vi "Calculate Mean Free Path.vi"(8 "error in (no error)":errorcluster, 11 "Gas Properties in":refnum<class "Gas Properties.lvclass">) -> (0 "error out":errorcluster, 2 "l (mm)":dbl, 3 "Gas Properties out":refnum<class "Gas Properties.lvclass">)   [LabVIEW 2015, in "Gas Properties.lvclass"]
uses:
  Gas Properties.lvclass
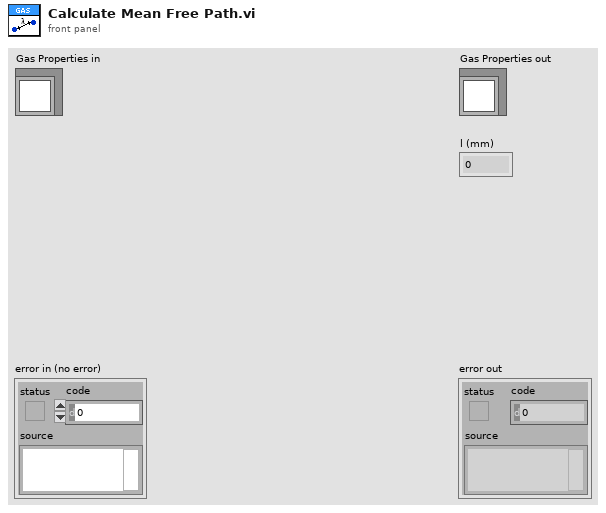
[diagram p1: front panel]
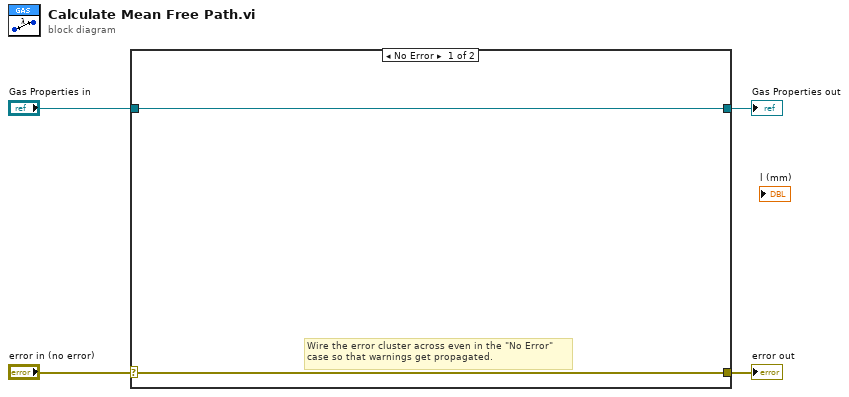
[diagram p0: block diagram]
diagram:
  n1 = case shown="No Error" "error in (no error)" {
    selector: "error in (no error)" -> [w5 w8]
    tunnel: [w5 w8] -> w3
    tunnel: [w6 w7] -> w1
    tunnel: "Gas Properties in" -> [w6 w7]
    frame No Error {
      # "Wire the error cluster across even in the \"No Error\"\ncase so that warnings get propagated."
    }
    frame Error {
    }
  }
  "error out" <- w3
  "Gas Properties out" <- w1
